vi "auxilary blocks.vi"() -> ()   [LabVIEW 2017]
uses:
  <vilib>/addons/Modulation/Analog/support/mod_Set Error Source.vi
  <vilib>/addons/Modulation/Digital/General/MT Generate Bits (Galois, Primitive Polynomial).vi
  <vilib>/Analysis/7linalg.llb/Create Special Real Matrix.vi
  <vilib>/Analysis/Matrix/Numeric/Conversions/Matrix To Array - RM.vi
  <vilib>/addons/Modulation/Digital/Support/Common/Validators/mod_Generate Filter Coefficients Validate.vi
  <vilib>/addons/Modulation/Digital/General/subVIs/mod_Generate Filter Coefficients.vi
  <vilib>/Analysis/2dsp.llb/Upsample (CDB).vi
  <vilib>/Analysis/3filter.llb/FIR Filter (CDB).vi
  <vilib>/addons/Modulation/niDMT.lvlib
  <vilib>/Analysis/NI_AALPro.lvlib
  <vilib>/Analysis/Matrix/NI_Matrix.lvlib
  <vilib>/Analysis/NI_AALBase.lvlib
  <vilib>/ptbypt/NI_PtbyPt.lvlib
panel:
  out "Параметры метрики":T1(array[cluster])
  out "permutation":i32[](array[numeric])=[0, 16, 32, 48, 64, 80, 96, 112, 128, 144, 160, 176, 192, 208, 224, 240, 256, 272, 288, 304, 320, 336, 352, 368, 1, 17, 33, 49, 65, 81, 97, 113, 129, 145, 161, 177, 193, 209, 225, 241, 257, 273, 289, 305, 321, 337, 353, 369, 2, 18, 34, 50, 66, 82, 98, 114, 130, 146, 162, 178, 194, 210, 226, 242, 258, 274, 290, 306, 322, 338, 354, 370, 3, 19, 35, 51, 67, 83, 99, 115, 131, 147, 163, 179, 195, 211, 227, 243, 259, 275, 291, 307, 323, 339, 355, 371, 4, 20, 36, 52, 68, 84, 100, 116, 132, 148, 164, 180, 196, 212, 228, 244, 260, 276, 292, 308, 324, 340, 356, 372, 5, 21, 37, 53, 69, 85, 101, 117, 133, 149, 165, 181, 197, 213, 229, 245, 261, 277, 293, 309, 325, 341, 357, 373, 6, 22, 38, 54, 70, 86, 102, 118, 134, 150, 166, 182, 198, 214, 230, 246, 262, 278, 294, 310, 326, 342, 358, 374, 7, 23, 39, 55, 71, 87, 103, 119, 135, 151, 167, 183, 199, 215, 231, 247, 263, 279, 295, 311, 327, 343, 359, 375, 8, 24, 40, 56, 72, 88, 104, 120, 136, 152, 168, 184, 200, 216, 232, 248, 264, 280, 296, 312, 328, 344, 360, 376, 9, 25, 41, 57, 73, 89, 105, 121, 137, 153, 169, 185, 201, 217, 233, 249, 265, 281, 297, 313, 329, 345, 361, 377, 10, 26, 42, 58, 74, 90, 106, 122, 138, 154, 170, 186, 202, 218, 234, 250, 266, 282, 298, 314, 330, 346, 362, 378, 11, 27, 43, 59, 75, 91, 107, 123, 139, 155, 171, 187, 203, 219, 235, 251, 267, 283, 299, 315, 331, 347, 363, 379, 12, 28, 44, 60, 76, 92, 108, 124, 140, 156, 172, 188, 204, 220, 236, 252, 268, 284, 300, 316, 332, 348, 364, 380, 13, 29, 45, 61, 77, 93, 109, 125, 141, 157, 173, 189, 205, 221, 237, 253, 269, 285, 301, 317, 333, 349, 365, 381, 14, 30, 46, 62, 78, 94, 110, 126, 142, 158, 174, 190, 206, 222, 238, 254, 270, 286, 302, 318, 334, 350, 366, 382, 15, 31, 47, 63, 79, 95, 111, 127, 143, 159, 175, 191, 207, 223, 239, 255, 271, 287, 303, 319, 335, 351, 367, 383]
  out "Выборка \nс канала":cdb
  in  "Выборка\nс передатчика":cdb format="%#.6g"
  out "Дискретизированная импульсная характеристика(коэффициенты) 2":dbl[](array[numeric]) caption="pulse shaping filter coefficients" format="%.2f"
  out "Импульсная характеристика":dbl[](graph)
  out "нечетные коэффициенты":dbl[](array[numeric])
  out "Четные коэффициенты":dbl[](array[numeric])
  out "ref signals":cdb[][](array[numeric])
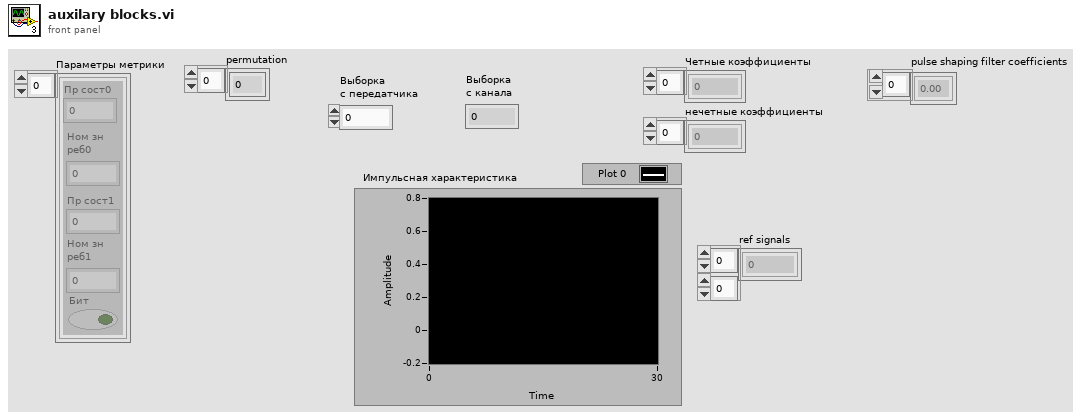
[diagram p1: front panel]
types:
  T1 = cluster{"Пр сост0":i32, "Ном зн\nреб0":i32, "Пр сост1":i32, "Ном зн\nреб1":i32, "Бит":bool}[]
  T2 = enum16{"none", "Raised Cosine", "Root Raised Cos", "Gaussian"}
  T3 = enum16{"FSK", "PSK", "QAM", "MSK", "PAM", "ASK", "CPM"}
  T4 = cluster{i32, i32, i32, i32, "lsb carry out":bool}
  T5 = typedef "NI_Matrix.lvlib/RealMatrix.ctl" = dbl[][]
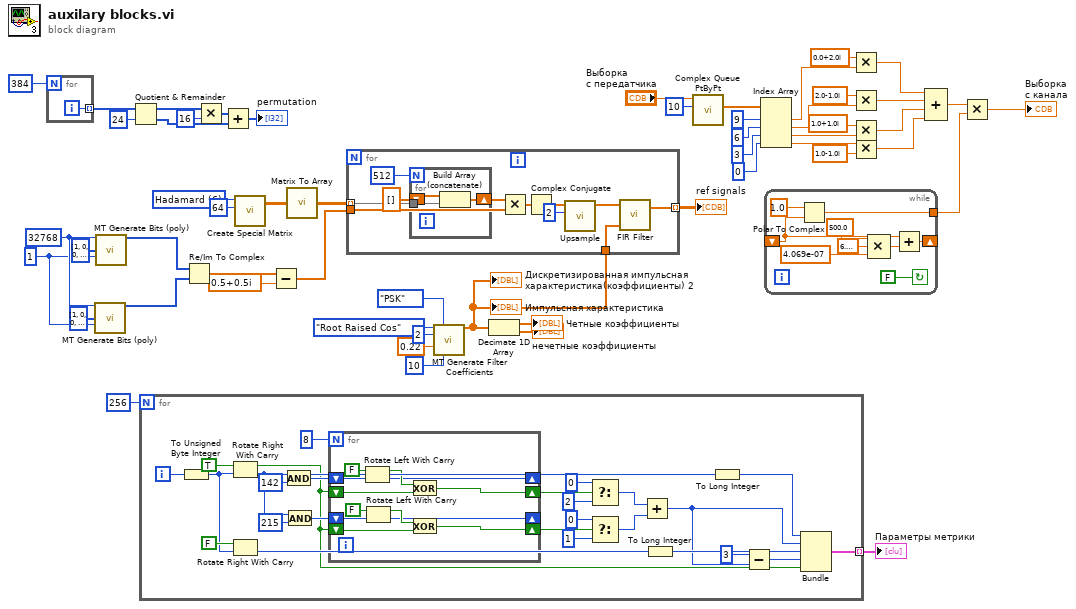
[diagram p0: block diagram]
diagram:
  w46 = 6 items=["Identity", "Diagonal", "Toeplitz", "Vandermonde", "Companion", "Hankel", "Hadamard", "Wilkinson", "Hilbert", "Inverse Hilbert", "Rosser", "Pascal"] ("matrix type")
  w49 = 1 ("seed in (0xD6BF7DF2)")
  w50 = 32768 ("total bits (128)")
  n1 = for {
    N: 384 -> [_]
    tunnel: [w55] -> w9 mode=indexing
    i -> [w55]
  }
  n2 = call-poly <vilib>:"MT Generate Bits (poly).vi"("total bits (128)"=w50, "specify primitive polynomial"=i8[] [1, 0, 0, 1, 1, 1, 1, 0, 0, 0, 1, 1, 1, 0, 0, 1], "seed in (0xD6BF7DF2)"=w49) -> ("output bit stream"=w53:i8[])  [unwired: 10 in, 2 out]
  n3 = call-poly <vilib>:"MT Generate Bits (poly).vi"("total bits (128)"=w50, "specify primitive polynomial"=i8[] [1, 0, 0, 0, 0, 1, 0, 1, 1, 1, 0, 0, 0, 1, 0, 1], "seed in (0xD6BF7DF2)"=w49) -> ("output bit stream"=w54:i8[])  [unwired: 10 in, 2 out]
  n4 = Quotient & Remainder(x=w9, y=24) -> (x-y*floor(x/y)=w7:i32[], floor(x/y)=w4:i32[])
  n5 = for {
    N: 256 -> [_]
    tunnel: [w60] -> w1 mode=indexing
    i -> [w66]
    n6 = To Unsigned Byte Integer(number=w66) -> (unsigned 8bit integer=w65:u8)
    n7 = Rotate Right With Carry(2:w65, 3:TRUE) -> (0:w62:u8, 1:w59:bool)
    n8 = Rotate Right With Carry(2:w65, 3:FALSE ("carry")) -> (0:w64:u8)  [unwired: 1 out]
    n9 = And(x=w62, y=u8 142) -> (x .and. y?=w78:u8)
    n10 = And(x=w62, y=u8 215) -> (x .and. y?=w77:u8)
    n11 = for {
      N: 8 -> [_]
      shift-right: [w88] -> w74
      shift-left: w59 -> [w87]
      shift-right: [w85] -> w69
      shift-left: w59 -> [w84]
      shift-right: [w83] -> _
      shift-left: w78 -> [w93]
      shift-right: [w82] -> _
      shift-left: w77 -> [w92]
      n12 = Rotate Left With Carry(2:w93, 3:FALSE ("carry")) -> (0:w83:u8, 1:w89:bool)
      n13 = Rotate Left With Carry(2:w92, 3:FALSE ("carry")) -> (0:w82:u8, 1:w86:bool)
      n14 = Exclusive Or(1:w87, 2:w89) -> (0:w88:bool)
      n15 = Exclusive Or(1:w84, 2:w86) -> (0:w85:bool)
    }
    n16 = Select(t=0, s=w74, f=2) -> (s? t:f=w68:i32)
    n17 = Select(t=0, s=w69, f=1) -> (s? t:f=w67:i32)
    n18 = Add(x=w68, y=w67) -> (x+y=w57:i32)
    n19 = To Long Integer(number=w64) -> (32bit integer=w63:i32)
    n20 = To Long Integer(number=w62) -> (32bit integer=w61:i32)
    n21 = Subtract(x=3, y=w57) -> (x-y=w58:i32)
    n22 = Bundle(w61, w57, w63, w58, "lsb carry out"=w59) -> (w60:T4)  [unwired: 1 in]
  }
  "Параметры метрики" <- w1
  n23 = Re/Im To Complex(1:w53, 2:w54) -> (0:w52:cdb[])
  n24 = Multiply(x=w7, y=16) -> (x*y=w5:i32[])
  n25 = Add(x=w5, y=w4) -> (x+y=→"permutation":i32[])
  n26 = call-poly <vilib>:"Create Special Matrix.vi"("matrix type"=w46, "matrix size"=64) -> ("Special Matrix"=w44:T5)  [unwired: 3 in, 1 out]
  n27 = Subtract(x=w52, y=cdb 0.5+0.5i) -> (x-y=w42:cdb[])
  n28 = call-poly <vilib>:"Matrix To Array.vi"("Real Matrix"=w44) -> ("Real 2D Array"=w43:dbl[][])
  n29 = call <vilib>:"MT Generate Filter Coefficients.vi"("pulse shaping filter (none)"=T2."Root Raised Cos", "modulation type"=T3."PSK", "pulse shaping samples per symbol (16)"=2, "filter parameter"=0.22, "filter length (symbols)"=10) -> ("pulse shaping filter coefficients"=w33:dbl[])  [unwired: 8 in, 2 out]
  "Импульсная характеристика" <- w33
  "Дискретизированная импульсная характеристика(коэффициенты) 2" <- w33
  n30 = for {
    tunnel: w43 -> [w104] mode=indexing
    tunnel: w42 -> [w100]
    tunnel: [w95] -> w41 mode=indexing
    tunnel: w33 -> [w94]
    n31 = for {
      N: 512 -> [_]
      tunnel: w104 -> [w107]
      shift-right: [w106] -> w101
      shift-left: dbl[] [] -> [w105]
      n32 = Build Array (concatenate)(w105, w107) -> (w106:dbl[])
    }
    n33 = Multiply(x=w101, y=w100) -> (x*y=w99:cdb[])
    n34 = Complex Conjugate(1:w99) -> (0:w96:cdb[])
    n35 = call-poly <vilib>:"Upsample.vi"("upsampling factor"=2, "X"=w96) -> ("Upsampled Array"=w97:cdb[])  [unwired: 8 in, 1 out]
    n36 = call-poly <vilib>:"FIR Filter.vi"("FIR Coefficients"=w94, "X"=w97) -> ("Filtered X"=w95:cdb[])  [unwired: 2 in, 1 out]
  }
  "ref signals" <- w41
  n37 = Decimate 1D Array(w33) -> (→"Четные коэффициенты":dbl[], →"нечетные коэффициенты":dbl[])
  n38 = call <vilib>:"Complex Queue PtByPt.vi"("sample length"=10, "input data point"="Выборка\nс передатчика") -> ("Current Queue"=w30:cdb[])  [unwired: 5 in, 4 out]
  n39 = Index Array(array=w30, index #1=9 ("index"), index #2=6 ("index"), index #3=3 ("index"), index #4=0 ("index")) -> (element #1=w25:cdb, element #2=w24:cdb, element #3=w23:cdb, element #4=w22:cdb)
  n40 = while {
    shift-right: [w111] -> _
    shift-left: _ -> [w110]
    tunnel: [w108] -> w15
    stop <- FALSE continue-if-true
    n41 = Polar To Complex(1:w110, 2:1.0 ("r")) -> (0:w108:cdb)
    n42 = Compound Arithmetic op=MULTIPLY(500.0, 6.283185307179586, 4.069e-07 ("value")) -> (w112:dbl)
    n43 = Add(x=w110, y=w112) -> (x+y=w111:dbl)
  }
  n44 = Multiply(x=cdb 0.0+2.0i, y=w25) -> (x*y=w17:cdb)
  n45 = Multiply(x=cdb 2.0-1.0i, y=w24) -> (x*y=w13:cdb)
  n46 = Multiply(x=cdb 1.0+1.0i, y=w23) -> (x*y=w12:cdb)
  n47 = Multiply(x=w22, y=cdb 1.0-1.0i) -> (x*y=w11:cdb)
  n48 = Compound Arithmetic op=ADD(w17, w13, w12, w11) -> (w16:cdb)
  n49 = Multiply(x=w16, y=w15) -> (x*y=→"Выборка \nс канала":cdb)
